vi "Get References.vi"() -> (2 "DMM resource name":refnum<visa-resource-name>="GPIB0::8::INSTR", 3 "ARB resource name":refnum<visa-resource-name>="GPIB0::7::INSTR", 4 "SMU1 resource name":refnum<visa-resource-name>="GPIB0::9::INSTR", 6 "SMU2 resource name":refnum<visa-resource-name>="GPIB0::10::INSTR", 8 "SMU3 resource name":refnum<visa-resource-name>="GPIB0::6::INSTR", 10 "DIG1 resource name":refnum<k15>="PXI1Slot6", 12 "MICS Dongle resource name":refnum<visa-resource-name>="COM5", 13 "Tegam2 resource name":refnum<visa-resource-name>="PXI4::14::INSTR", 14 "Tegam1 resource name":refnum<visa-resource-name>="PXI4::12::INSTR", 15 "DIG2 resource name":refnum<k15>="PXI1Slot4")   [LabVIEW 2010]
doc: "This function provides a complete test set list of instrument resource names (addresses)."
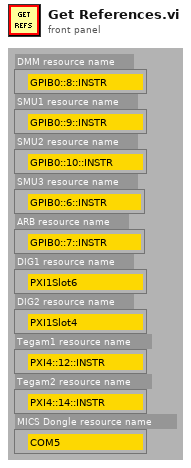
[diagram p1: front panel]
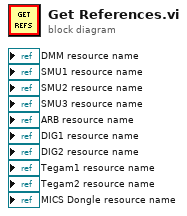
[diagram p0: block diagram]
diagram:
